vi "trash_Write Last Value.vi"(8 "error in (no error)":errorcluster, 10 "Last Value":variant, 11 "CIFChannels in":refnum<class "CIFChannels.lvclass">) -> (0 "error out":errorcluster, 3 "CIFChannels out":refnum<class "CIFChannels.lvclass">)   [LabVIEW 2021]
uses:
  CIFChannels.lvclass/CIFChannels.ctl
  CIFChannels.lvclass
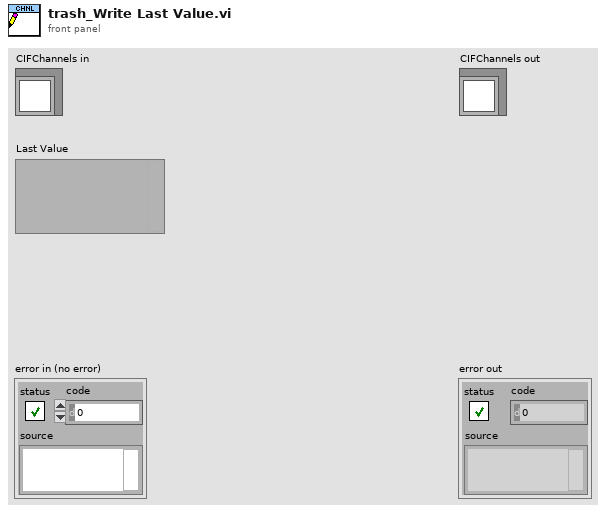
[diagram p1: front panel]
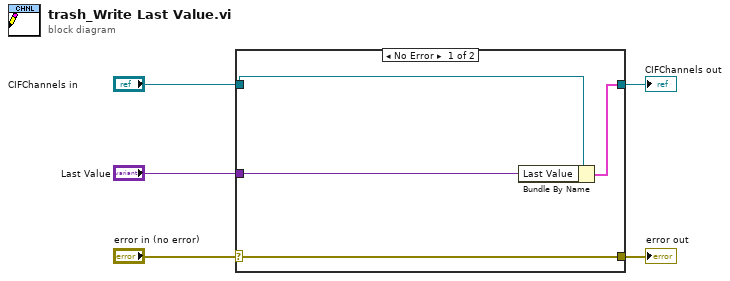
[diagram p0: block diagram]
diagram:
  n1 = case shown="No Error" "error in (no error)" {
    selector: "error in (no error)" -> [w9 w10]
    tunnel: [w9 w10] -> w4
    tunnel: [w7 w11] -> w2
    tunnel: "CIFChannels in" -> [w8 w11]
    tunnel: "Last Value" -> [w6 _]
    frame No Error {
      n2 = Bundle By Name(cluster=w8, "Last Value"=w6) -> (w7:cluster{})
    }
    frame Error {
    }
  }
  "error out" <- w4
  "CIFChannels out" <- w2
